vi "Report Num Array Command.vi"(7 "Level (Info)":T2=enum."Info", 8 "error in (no error)":errorcluster, 10 "Command":T1[](array[typedef]), 11 "Module in":refnum<class "Module.lvclass">) -> (0 "error out":errorcluster, 3 "Module out":refnum<class "Module.lvclass">)   [LabVIEW 2020, in "Volatus.lvlib" / "Module.lvclass"]
uses:
  Module.lvclass
  Module.lvclass/Module.ctl
  Event Level.ctl
  Volatus.lvlib
  messages/CmdAnalog/Data.ctl
  messages/CmdAnalog/CmdAnalog.lvlib
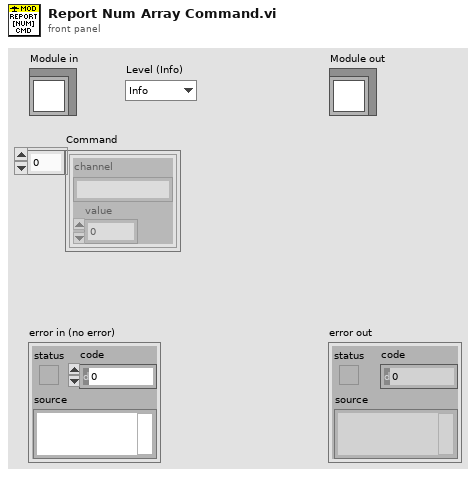
[diagram p1: front panel]
types:
  T1 = typedef "CmdAnalog.lvlib/Data.ctl" = cluster{"channel":string, "value":dbl}
  T2 = typedef "Volatus.lvlib/Event Level.ctl" = enum16{"Debug", "Info", "Warning", "Error"}
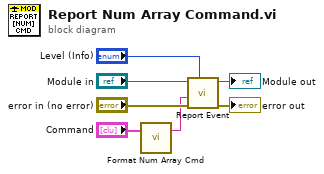
[diagram p0: block diagram]
diagram:
  n1 = call "Format Num Array Cmd.vi"("Command"="Command") -> ("String"=w1:string)  [unwired: 6 in]
  n2 = call "Report Event.vi"("Level (Info)"="Level (Info)", "error in (no error)"="error in (no error)", "Message"=w1, "Module in"="Module in") -> ("error out"=→"error out":errorcluster, "Module out"=→"Module out":refnum<class "Module.lvclass">)  [unwired: 6 in]
